vi "Drive Test.vi"(9 "Progress":string, 10 "ProgressText":string) -> (2 "EndTestText":string)   [LabVIEW 2012]
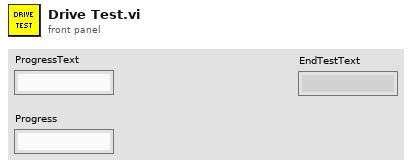
[diagram p1: front panel]
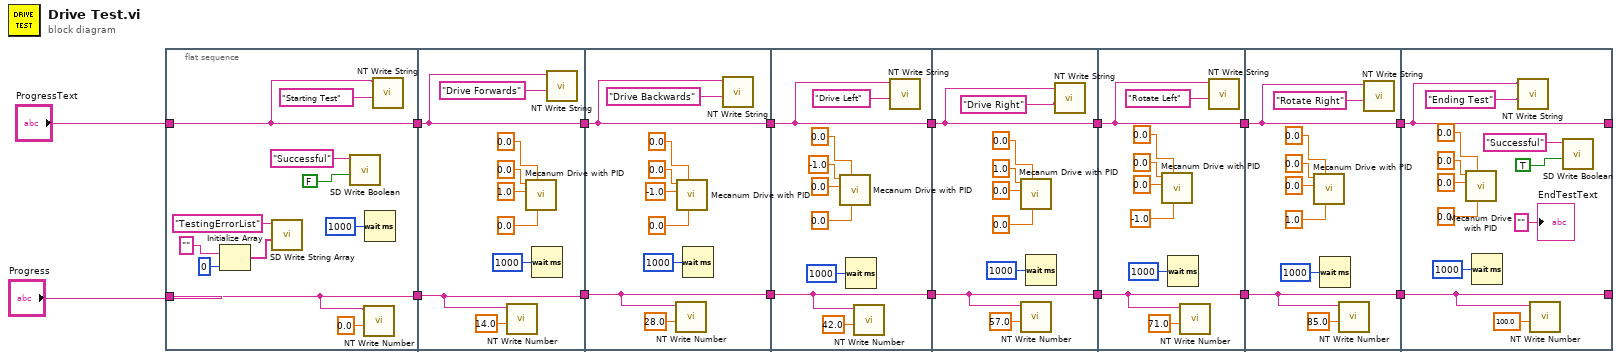
[diagram p0: block diagram]
diagram:
  n1 = flat-sequence {
    tunnel: "ProgressText" -> [w23]
    tunnel: "Progress" -> [w26]
    tunnel: [w23] -> w15
    tunnel: [w26] -> w14
    tunnel: w15 -> [w29]
    tunnel: w14 -> [w31]
    tunnel: [w29] -> w12
    tunnel: [w31] -> w11
    tunnel: w12 -> [w37]
    tunnel: w11 -> [w40]
    tunnel: [w37] -> w10
    tunnel: [w40] -> w9
    tunnel: w10 -> [w47]
    tunnel: w9 -> [w49]
    tunnel: [w47] -> w8
    tunnel: [w49] -> w7
    tunnel: w8 -> [w56]
    tunnel: w7 -> [w58]
    tunnel: [w56] -> w6
    tunnel: [w58] -> w5
    tunnel: w6 -> [w65]
    tunnel: w5 -> [w67]
    tunnel: [w65] -> w4
    tunnel: [w67] -> w3
    tunnel: w4 -> [w74]
    tunnel: w3 -> [w76]
    tunnel: [w74] -> w2
    tunnel: [w76] -> w1
    tunnel: [w87] -> _
    tunnel: [w85] -> _
    tunnel: w2 -> [w85]
    tunnel: w1 -> [w87]
    frame #0 {
      n2 = Initialize Array("", 0 ("dimension size")) -> (w18:string[])
      n3 = call <vilib>:"SD Write String Array.vi"("String Array"=w18, "Name"="TestingErrorList") -> ()  [unwired: 8 in, 2 out]
      n4 = call <vilib>:"SD Write Boolean.vi"("Boolean"=FALSE, "Name"="Successful") -> ()  [unwired: 8 in, 2 out]
      n5 = call <vilib>:"NT Write Number.vi"("Numeric"=0.0, "Name"=w26) -> ()  [unwired: 9 in, 1 out]
      n6 = Wait (ms)(milliseconds to wait=u32 1000) -> ()  [unwired: 1 out]
      n7 = call <vilib>:"NT Write String.vi"("String"="Starting Test", "Name"=w23) -> ()  [unwired: 9 in, 1 out]
    }
    frame #1 {
      n8 = call <vilib>:"NT Write Number.vi"("Numeric"=14.0, "Name"=w31) -> ()  [unwired: 9 in, 1 out]
      n9 = call "Mecanum Drive with PID.vi"("Rotation"=0.0, "MaxSpeed"=0.0 ("Gyro Angle"), "Y"=1.0, "X"=0.0) -> ()  [unwired: 8 in]
      n10 = Wait (ms)(milliseconds to wait=u32 1000) -> ()  [unwired: 1 out]
      n11 = call <vilib>:"NT Write String.vi"("String"="Drive Forwards", "Name"=w29) -> ()  [unwired: 9 in, 1 out]
    }
    frame #2 {
      n12 = call <vilib>:"NT Write Number.vi"("Numeric"=28.0, "Name"=w40) -> ()  [unwired: 9 in, 1 out]
      n13 = call "Mecanum Drive with PID.vi"("Rotation"=0.0, "MaxSpeed"=0.0 ("Gyro Angle"), "Y"=-1.0, "X"=0.0) -> ()  [unwired: 8 in]
      n14 = Wait (ms)(milliseconds to wait=u32 1000) -> ()  [unwired: 1 out]
      n15 = call <vilib>:"NT Write String.vi"("String"="Drive Backwards", "Name"=w37) -> ()  [unwired: 9 in, 1 out]
    }
    frame #3 {
      n16 = call "Mecanum Drive with PID.vi"("Rotation"=0.0, "MaxSpeed"=0.0 ("Gyro Angle"), "Y"=0.0, "X"=-1.0) -> ()  [unwired: 8 in]
      n17 = Wait (ms)(milliseconds to wait=u32 1000) -> ()  [unwired: 1 out]
      n18 = call <vilib>:"NT Write Number.vi"("Numeric"=42.0, "Name"=w49) -> ()  [unwired: 9 in, 1 out]
      n19 = call <vilib>:"NT Write String.vi"("String"="Drive Left", "Name"=w47) -> ()  [unwired: 9 in, 1 out]
    }
    frame #4 {
      n20 = call "Mecanum Drive with PID.vi"("Rotation"=0.0, "MaxSpeed"=0.0 ("Gyro Angle"), "Y"=0.0, "X"=1.0) -> ()  [unwired: 8 in]
      n21 = call <vilib>:"NT Write Number.vi"("Numeric"=57.0, "Name"=w58) -> ()  [unwired: 9 in, 1 out]
      n22 = Wait (ms)(milliseconds to wait=u32 1000) -> ()  [unwired: 1 out]
      n23 = call <vilib>:"NT Write String.vi"("String"="Drive Right", "Name"=w56) -> ()  [unwired: 9 in, 1 out]
    }
    frame #5 {
      n24 = call "Mecanum Drive with PID.vi"("Rotation"=-1.0, "MaxSpeed"=0.0 ("Gyro Angle"), "Y"=0.0, "X"=0.0) -> ()  [unwired: 8 in]
      n25 = Wait (ms)(milliseconds to wait=u32 1000) -> ()  [unwired: 1 out]
      n26 = call <vilib>:"NT Write Number.vi"("Numeric"=71.0, "Name"=w67) -> ()  [unwired: 9 in, 1 out]
      n27 = call <vilib>:"NT Write String.vi"("String"="Rotate Left", "Name"=w65) -> ()  [unwired: 9 in, 1 out]
    }
    frame #6 {
      n28 = call "Mecanum Drive with PID.vi"("Rotation"=1.0, "MaxSpeed"=0.0 ("Gyro Angle"), "Y"=0.0, "X"=0.0) -> ()  [unwired: 8 in]
      n29 = Wait (ms)(milliseconds to wait=u32 1000) -> ()  [unwired: 1 out]
      n30 = call <vilib>:"NT Write Number.vi"("Numeric"=85.0, "Name"=w76) -> ()  [unwired: 9 in, 1 out]
      n31 = call <vilib>:"NT Write String.vi"("String"="Rotate Right", "Name"=w74) -> ()  [unwired: 9 in, 1 out]
    }
    frame #7 {
      n32 = call "Mecanum Drive with PID.vi"("Rotation"=0.0, "MaxSpeed"=0.0 ("Gyro Angle"), "Y"=0.0, "X"=0.0) -> ()  [unwired: 8 in]
      n33 = Wait (ms)(milliseconds to wait=u32 1000) -> ()  [unwired: 1 out]
      n34 = call <vilib>:"NT Write String.vi"("String"="Ending Test", "Name"=w85) -> ()  [unwired: 9 in, 1 out]
      n35 = call <vilib>:"NT Write Number.vi"("Numeric"=100.0, "Name"=w87) -> ()  [unwired: 9 in, 1 out]
      n36 = call <vilib>:"SD Write Boolean.vi"("Boolean"=TRUE, "Name"="Successful") -> ()  [unwired: 8 in, 2 out]
      "EndTestText" <- "" ("EndTestText")
    }
  }
